vi "State Machine.vi"(0 "private data":T1={"instruction target"=refnum, "channels"=[], "measure state"=enum."Uninitialized", "rx output divider"=enum."1", "equalization mode"=enum."DFE", "rx internal data width"=enum."32 Bit", "BER floor"=0.0, "number of points completed"=0, "rx output divider configured?"=FALSE, "equalization mode configured?"=FALSE, "rx data width configured?"=FALSE}, 5 "requested number of new points":i32, 7 "timeout (100 ms)":dbl=0.1, 11 "error in":errorcluster) -> (4 "private data out":T1={"instruction target"=refnum, "channels"=[], "measure state"=enum."Uninitialized", "rx output divider"=enum."1", "equalization mode"=enum."DFE", "rx internal data width"=enum."32 Bit", "BER floor"=0.0, "number of points completed"=0, "rx output divider configured?"=FALSE, "equalization mode configured?"=FALSE, "rx data width configured?"=FALSE}, 6 "retrieved number of new points":i32, 8 "last point measured?":bool, 14 "timed out?":bool, 15 "error out":errorcluster)   [LabVIEW 2015, in "niHighSpeedSerial Eye Scan v1 Host.lvclass"]
doc: "Manages the state of the Eye Scan engine and handles storing of completed measurements and advancing to measure the next point in the scan.\n\n<B>Input Parameters</B>\n\n<B>private data</B> is the class private data input into the VI.\n\n<B>private data.instruction target</B> is the instruction target to use when communicating with the FPGA.\n\n<B>private data.channels</B> is the array of channel information.\n\n<B>private data.channels.instance</B> is the instance of the channel.\n\n<B>private data.channels.channel</B> is the channel object for a particular channel instance.\n\n<B>private data.channels.point iterator</B> is the point iterator which stores the channel's measured points and controls which point to measure next.\n\n<B>private data.measure state</B> maintains the internal state of the Eye Scan class.\nenum values: Uninitialized,Initialized,Ready,Measuring,Finished,Aborted\n\n<B>private data.rx output divider</B> represents the configuration of the receiver output divider. This should match the values configured with RXRATE and RXOUT_DIV.\nenum values: 1,2,4,8,16\n\n<B>private data.equalization mode</B> indicates the Equalization Mode that the lane is using.\nenum values: DFE,LPM\n\n<B>private data.data width</B> is the data width (in bits) of the receiver lane.\nenum values: 16 Bit,20 Bit,32 Bit,40 Bit\n\n<B>private data.BER floor</B> is the minimum Bit Error Rate which may be computed.\n\n<B>private data.number of points completed</B> is the number of points that have been completed so far by Eye Scan.\n\n<B>private data.rx output divider configured?</B> is true if you have configured the RX Output Divider.\n\n<B>private data.equalization mode configured?</B> is true if you have configured the Equalization Mode\n\n<B>private data.data width configured?</B> is true if you have configured the Data Width.\n\n<B>requested number of new points</B> The number of new points to return, assuming that timeout is not reached, the entire scan doesn't complete, and no errors occur.\n\n<B>timeout (100 ms)</B> The amount of time (in seconds) before timing timing out.\nSpecifying '-1' prevents 'timed out' from ever returning true.\n\n<B>error in</B> describes error conditions that occur before this node runs. This input provides standard 'error in' functionality.\n\n<B>Output Parameters</B>\n\n<B>private data out</B> is the class private data output from the VI.\n\n<B>private data out.instruction target</B> is the instruction target to use when communicating with the FPGA.\n\n<B>private data out.channels</B> is the array of channel information.\n\n<B>private data out.channels.instance</B> is the instance of the channel.\n\n<B>private data out.channels.channel</B> is the channel object for a particular channel instance.\n\n<B>private data out.channels.point iterator</B> is the point iterator which stores the channel's measured points and controls which point to measure next.\n\n<B>private data out.measure state</B> maintains the internal state of the Eye Scan class.\nenum values: Uninitialized,Initialized,Ready,Measuring,Finished,Aborted\n\n<B>private data out.rx output divider</B> represents the configuration of the receiver output divider. This should match the values configured with RXRATE and RXOUT_DIV.\nenum values: 1,2,4,8,16\n\n<B>private data out.equalization mode</B> indicates the Equalization Mode that the lane is using.\nenum values: DFE,LPM\n\n<B>private data out.data width</B> is the data width (in bits) of the receiver lane.\nenum values: 16 Bit,20 Bit,32 Bit,40 Bit\n\n<B>private data out.BER floor</B> is the minimum Bit Error Rate which may be computed.\n\n<B>private data out.number of points completed</B> is the number of points that have been completed so far by the Eye Scan algorithm.\n\n<B>private data out.rx output divider configured?</B> is true if you have configured the RX Output Divider.\n\n<B>private data out.equalization mode configured?</B> is true if you have configured the Equalization Mode.\n\n<B>private data out.data width configured?</B> is true if you have configured the Data Width.\n\n<B>retrieved number of new points</B> The number of new points that were retrieved in this call to Measure.\n\n<B>last point measured?</B> returns true if Eye Scan has completed measuring all points that it was configured to measure.\n\n<B>timed out?</B> returns true if at least 'timeout' amount of time has passed.\n\n<B>error out</B> contains error information. This output provides standard 'error out' functionality."
uses:
  <instrlib>/niHighSpeedSerial/Eye Scan/v1/Host/Eye Scan/niHighSpeedSerial Eye Scan v1 Host.lvclass
  <instrlib>/niHighSpeedSerial/Eye Scan/v1/Host/Eye Scan/Private/Private Data.ctl
  <instrlib>/_niInstr/Instruction Framework/v1/Host/Instruction Target/niInstr Instruction Target v1 Host.lvclass
  <instrlib>/niHighSpeedSerial/Eye Scan/v1/Host/Impl/Eye Scan Point Iterator/niHighSpeedSerial Eye Scan Point Iterator v1 Host.lvclass
  <instrlib>/niHighSpeedSerial/Eye Scan/v1/Host/Eye Scan/Private/Channel Data.ctl
  <instrlib>/niHighSpeedSerial/Eye Scan/v1/Host/Impl/Single Point/niHighSpeedSerial Eye Scan Single Point v1 Host.lvclass
  <instrlib>/niHighSpeedSerial/Eye Scan/v1/Host/Eye Scan/Private/Measure State.ctl
  <instrlib>/niHighSpeedSerial/Eye Scan/v1/Host/Common/Public/RX Output Divider.ctl
  <instrlib>/niHighSpeedSerial/Eye Scan/v1/Host/Common/Public/Equalization Mode.ctl
  <instrlib>/niHighSpeedSerial/Eye Scan/v1/Host/Common/Public/Data Width.ctl
  <instrlib>/niHighSpeedSerial/Eye Scan/v1/Host/Common/niHighSpeedSerial Eye Scan Common v1 Host.lvlib
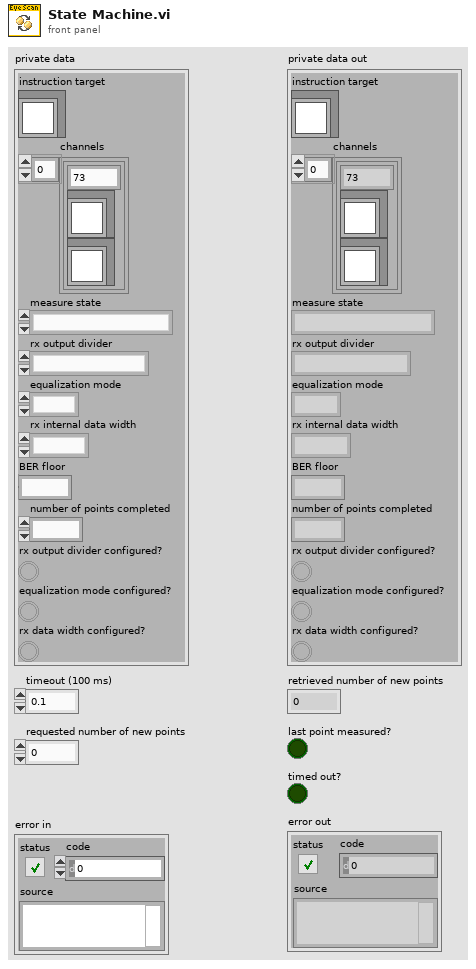
[diagram p1: front panel]
types:
  T1 = typedef "niHighSpeedSerial Eye Scan v1 Host.lvclass/Private Data.ctl" = cluster{"instruction target":refnum<class "niInstr Instruction Target v1 Host.lvclass">, "channels":T2[], "measure state":T3, "rx output divider":T4, "equalization mode":T5, "rx internal data width":T6, "BER floor":dbl, "number of points completed":i32, "rx output divider configured?":bool, "equalization mode configured?":bool, "rx data width configured?":bool}
  T2 = typedef "niHighSpeedSerial Eye Scan v1 Host.lvclass/Channel Data.ctl" = cluster{"instance":u8, "channel":refnum<class "niHighSpeedSerial Eye Scan Single Point v1 Host.lvclass">, "point iterator":refnum<class "niHighSpeedSerial Eye Scan Point Iterator v1 Host.lvclass">}
  T3 = typedef "niHighSpeedSerial Eye Scan v1 Host.lvclass/Measure State.ctl" = enum16{"Uninitialized", "Initialized", "Ready", "Measuring", "Finished", "Aborted"}
  T4 = typedef "niHighSpeedSerial Eye Scan Common v1 Host.lvlib/RX Output Divider.ctl" = enum16{"1", "2", "4", "8", "16"}
  T5 = typedef "niHighSpeedSerial Eye Scan Common v1 Host.lvlib/Equalization Mode.ctl" = enum16{"DFE", "LPM"}
  T6 = typedef "niHighSpeedSerial Eye Scan Common v1 Host.lvlib/Data Width.ctl" = enum16{"16 Bit", "20 Bit", "32 Bit", "40 Bit"}
  T7 = typedef "niHighSpeedSerial Eye Scan Common v1 Host.lvlib/Point Offsets.ctl" = cluster{"horizontal offset":i16, "vertical offset":i8}
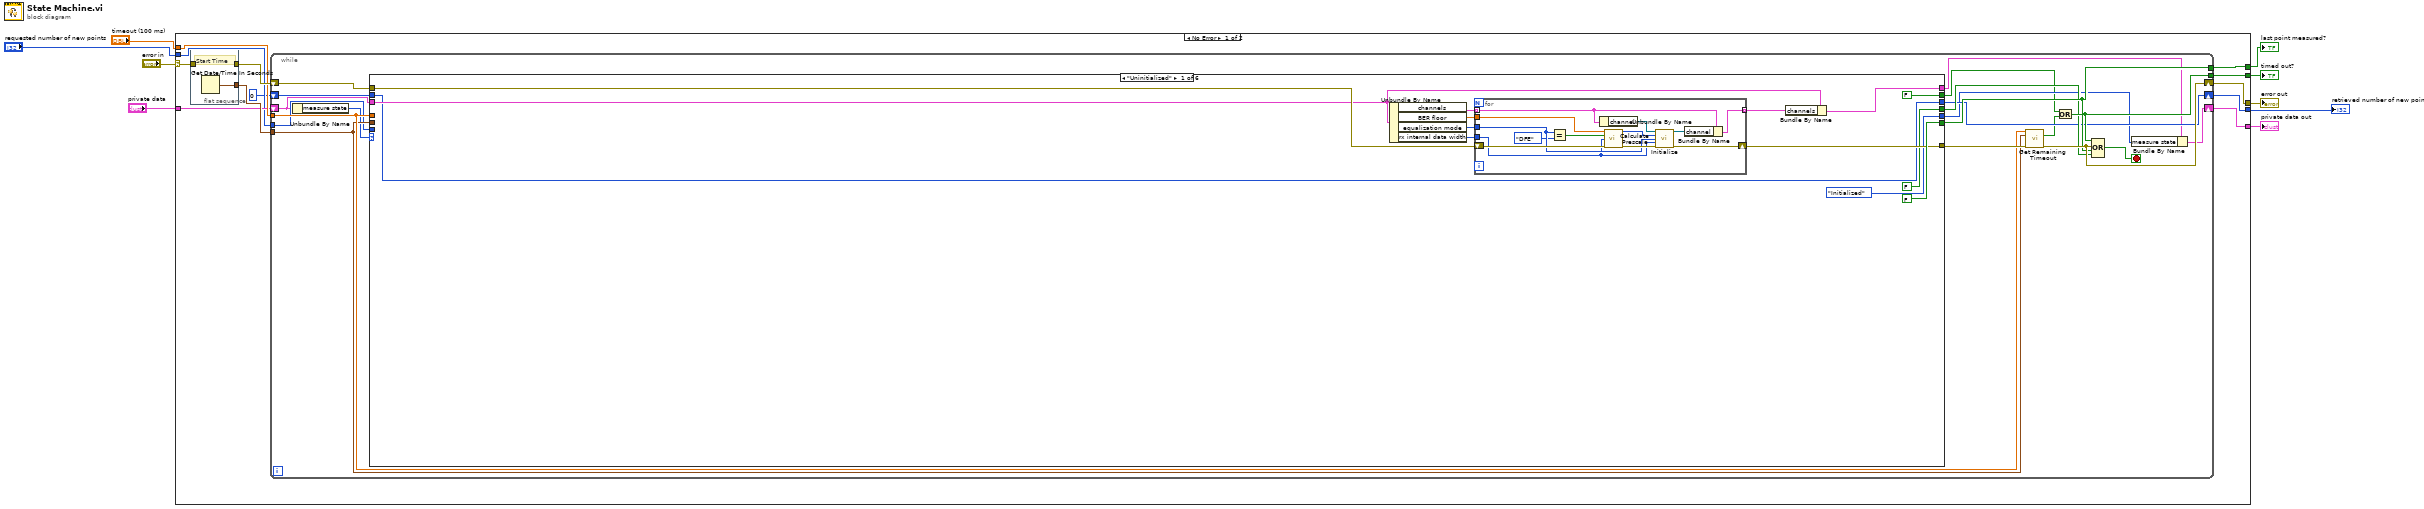
[diagram p0: block diagram]
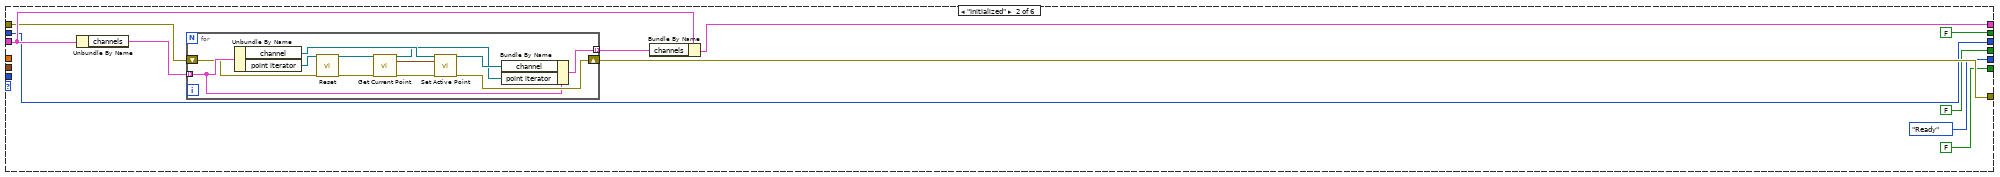
[diagram p2: hidden frame]
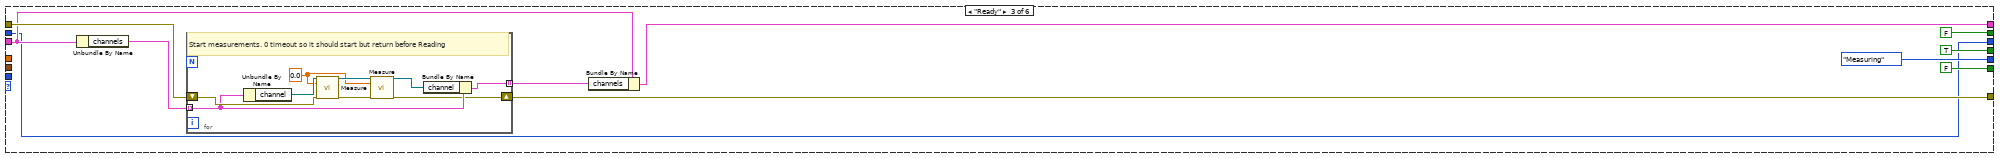
[diagram p3: hidden frame]
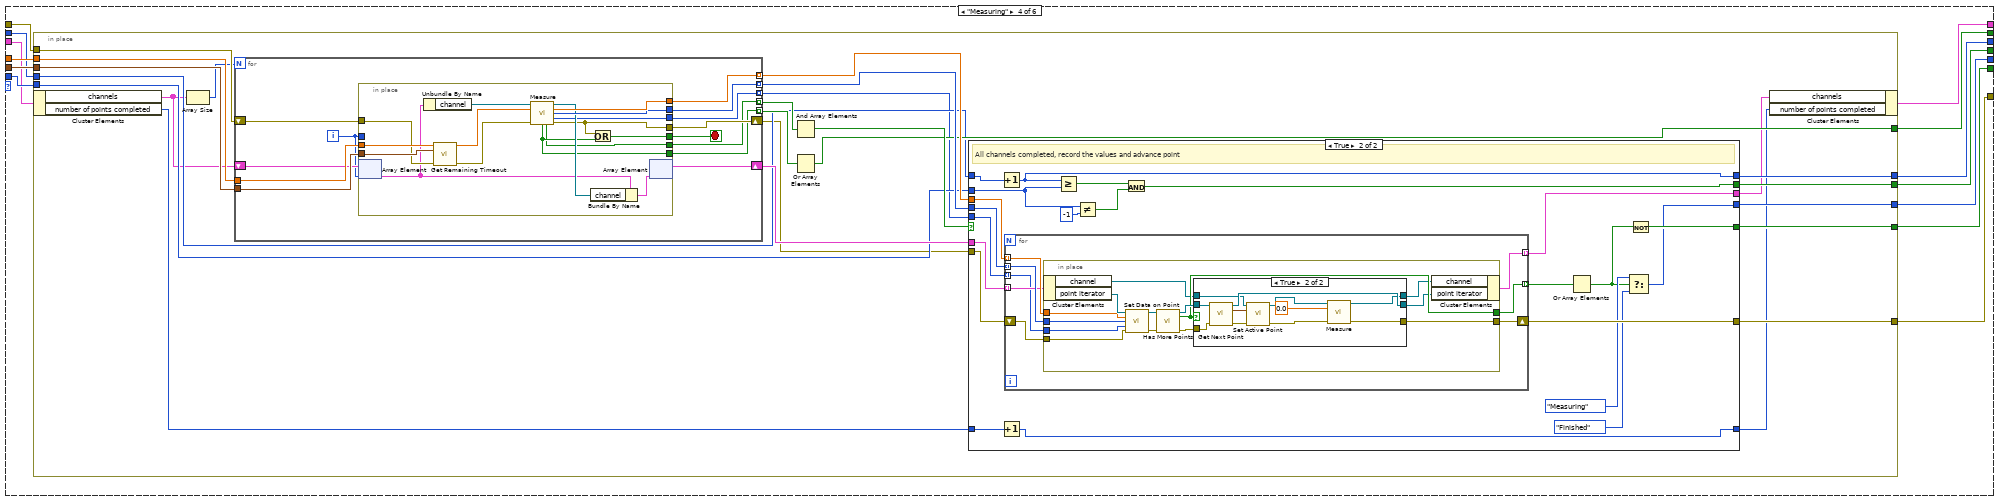
[diagram p4: hidden frame]
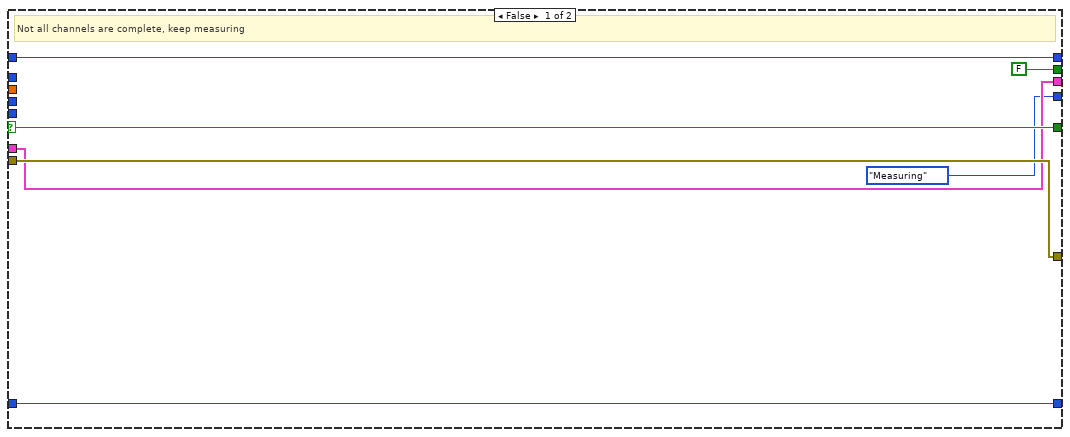
[diagram p5: hidden frame]
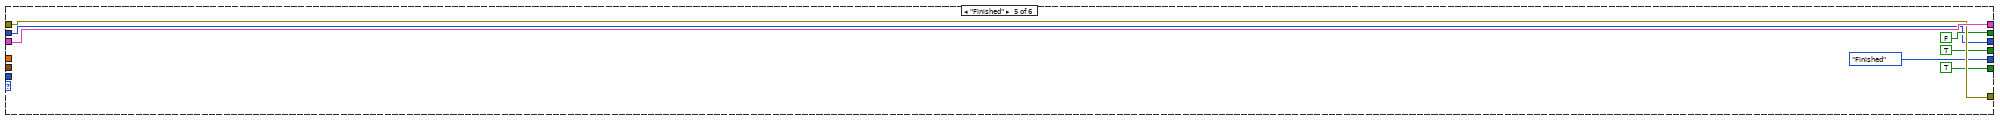
[diagram p7: hidden frame]
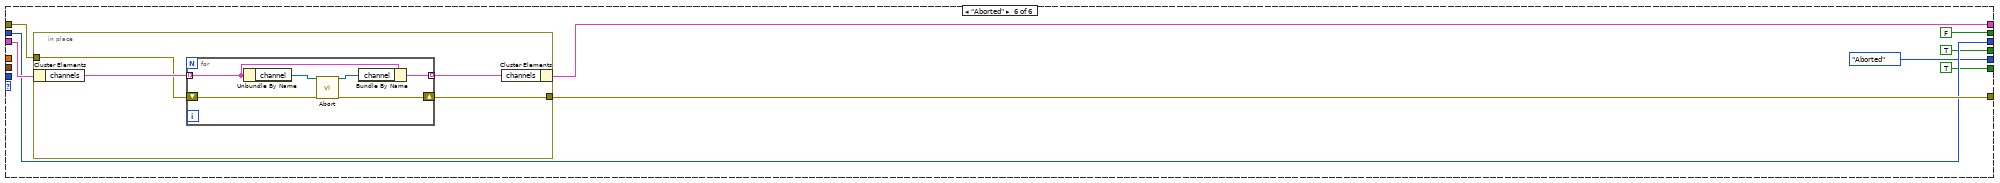
[diagram p8: hidden frame]
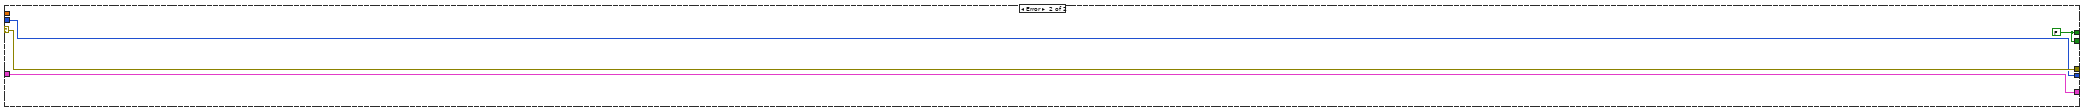
[diagram p9: hidden frame]
diagram:
  n1 = case shown="No Error" "error in" {
    selector: "error in" -> [w20 w272]
    tunnel: "timeout (100 ms)" -> [w18 _]
    tunnel: [w10 w273] -> w7
    tunnel: "private data" -> [w15 w273]
    tunnel: [w16 w272] -> w5
    tunnel: [w17 w271] -> w4
    tunnel: [w14 w271] -> w3
    tunnel: "requested number of new points" -> [w13 w270]
    tunnel: [w11 w270] -> w1
    frame No Error {
      n2 = flat-sequence {
        tunnel: w20 -> [w269]
        tunnel: [w269] -> w19
        tunnel: [w268] -> w21
        frame #0 {
          # "Start Time"
          n3 = Get Date/Time In Seconds() -> (seconds since 1Jan1904=w268:timestamp)
        }
      }
      n4 = while {
        tunnel: w21 -> [w32]
        shift-right: [w37] -> w16
        shift-left: w19 -> [w40]
        tunnel: w18 -> [w33]
        tunnel: [w36] -> w17
        tunnel: [w35] -> w14
        tunnel: w13 -> [w31]
        shift-right: [w29] -> w11
        shift-left: 0 ("Requested Number of Points") -> [w30]
        shift-right: [w24] -> w10
        shift-left: w15 -> [w28]
        stop <- w38 stop-if-true
        n5 = Unbundle By Name(w28) -> ("measure state"=w27:T3)
        n6 = case shown="\"Uninitialized\"" w27 {
          tunnel: w40 -> [w52 w68 w96 w121 w247 w256]
          tunnel: [w51 w77 w95 w119 w247 w255] -> w39
          tunnel: [FALSE ("done") FALSE ("done") FALSE ("done") w120 TRUE ("done") TRUE ("done")] -> w36
          tunnel: [FALSE ("done") FALSE ("done") FALSE ("done") w117 FALSE ("done") FALSE ("done")] -> w22
          tunnel: w28 -> [w49 w72 w94 w112 w248 w257]
          tunnel: [Measure_State."Initialized" ("Measure State") Measure_State."Ready" ("Measure State") Measure_State."Measuring" ("Measure State") w118 Measure_State."Finished" ("Measure State") Measure_State."Aborted" ("Measure State")] -> w25
          tunnel: [w48 w71 w92 w111 w248 w249] -> w26
          tunnel: [FALSE ("done") FALSE ("done") TRUE ("done") w113 TRUE ("done") TRUE ("done")] -> w34
          tunnel: w33 -> [_ _ _ w123 _ _]
          tunnel: w32 -> [_ _ _ w122 _ _]
          tunnel: w31 -> [_ _ _ w115 _ _]
          tunnel: w30 -> [w44 w69 w91 w116 w242 w254]
          tunnel: [w44 w69 w91 w114 w242 w254] -> w29
          frame "Uninitialized" {
            n7 = Unbundle By Name(w49) -> ("channels"=w53:T2[], "BER floor"=w43:dbl, "equalization mode"=w42:T5, "rx internal data width"=w41:T6)
            n8 = for {
              tunnel: w53 -> [w63] mode=indexing
              shift-right: [w67] -> w51
              shift-left: w52 -> [w61]
              tunnel: [w65] -> w47 mode=indexing
              tunnel: w43 -> [w62]
              tunnel: w42 -> [w58]
              tunnel: w41 -> [w55]
              n9 = Equal?(x=w58, y=Equalization_Mode."DFE") -> (x = y?=w56:bool)
              n10 = Unbundle By Name(w63) -> ("channel"=w66:refnum<class "niHighSpeedSerial Eye Scan Single Point v1 Host.lvclass">)
              n11 = call <instrlib>:"Calculate Prescale.vi"("minimum BER"=w62, "in DFE mode?"=w56, "receiver data width"=w55, "error in"=w61) -> ("prescale"=w59:u8, "error out"=w60:errorcluster)  [unwired: 10 in]
              n12 = call-dynamic "Initialize.vi"("eye scan single point"=w66, "prescale"=w59, "equalization mode"=w58, "receiver data width"=w55, "error in"=w60) -> ("eye scan single point out"=w64:refnum<class "niHighSpeedSerial Eye Scan Single Point v1 Host.lvclass">, "error out"=w67:errorcluster)  [unwired: 9 in]
              n13 = Bundle By Name(cluster=w63, "channel"=w64) -> (w65:T2)
            }
            n14 = Bundle By Name(cluster=w49, "channels"=w47) -> (w48:T1)
          }
          frame "Initialized" {
            n15 = Unbundle By Name(w72) -> ("channels"=w78:T2[])
            n16 = for {
              tunnel: w78 -> [w88] mode=indexing
              shift-right: [w90] -> w77
              shift-left: w68 -> [w85]
              tunnel: [w86] -> w70 mode=indexing
              n17 = Unbundle By Name(w88) -> ("channel"=w89:refnum<class "niHighSpeedSerial Eye Scan Single Point v1 Host.lvclass">, "point iterator"=w84:refnum<class "niHighSpeedSerial Eye Scan Point Iterator v1 Host.lvclass">)
              n18 = call-dynamic "Reset.vi"("eye scan point iterator"=w84, "error in"=w85) -> ("eye scan point iterator out"=w83:refnum<class "niHighSpeedSerial Eye Scan Point Iterator v1 Host.lvclass">, "error out"=w82:errorcluster)  [unwired: 12 in]
              n19 = call-dynamic "Get Current Point.vi"("eye scan point iterator"=w83, "error in"=w82) -> ("eye scan point iterator out"=w81:refnum<class "niHighSpeedSerial Eye Scan Point Iterator v1 Host.lvclass">, "current point"=w80:T7, "error out"=w79:errorcluster)  [unwired: 11 in]
              n20 = call-dynamic "Set Active Point.vi"("eye scan single point"=w89, "active point"=w80, "error in"=w79) -> ("eye scan single point out"=w87:refnum<class "niHighSpeedSerial Eye Scan Single Point v1 Host.lvclass">, "error out"=w90:errorcluster)  [unwired: 11 in]
              n21 = Bundle By Name(cluster=w88, "channel"=w87, "point iterator"=w81) -> (w86:T2)
            }
            n22 = Bundle By Name(cluster=w72, "channels"=w70) -> (w71:T1)
          }
          frame "Ready" {
            n23 = Unbundle By Name(w94) -> ("channels"=w97:T2[])
            n24 = for {
              tunnel: w97 -> [w108] mode=indexing
              shift-right: [w103] -> w95
              shift-left: w96 -> [w110]
              tunnel: [w107] -> w93 mode=indexing
              w102 = 0.0 ("Timeout (100 ms)")
              # "Start measurements. 0 timeout so it should start but return before Reading"
              n25 = Unbundle By Name(w108) -> ("channel"=w109:refnum<class "niHighSpeedSerial Eye Scan Single Point v1 Host.lvclass">)
              n26 = call-dynamic "Measure.vi"("eye scan single point"=w109, "timeout (100 ms)"=w102, "error in"=w110) -> ("eye scan single point out"=w106:refnum<class "niHighSpeedSerial Eye Scan Single Point v1 Host.lvclass">, "error out"=w105:errorcluster)  [unwired: 6 in, 5 out]
              n27 = call-dynamic "Measure.vi"("eye scan single point"=w106, "timeout (100 ms)"=w102, "error in"=w105) -> ("eye scan single point out"=w104:refnum<class "niHighSpeedSerial Eye Scan Single Point v1 Host.lvclass">, "error out"=w103:errorcluster)  [unwired: 6 in, 5 out]
              n28 = Bundle By Name(cluster=w108, "channel"=w104) -> (w107:T2)
            }
            n29 = Bundle By Name(cluster=w94, "channels"=w93) -> (w92:T1)
          }
          frame "Measuring" {
            n30 = in-place {
              in-place-border: w123 -> [w147]
              in-place-border: w122 -> [w146]
              in-place-border: w121 -> [w145]
              in-place-border: [w139] -> w120
              in-place-border: [w137] -> w119
              in-place-border: [w136] -> w118
              in-place-border: [w135] -> w117
              in-place-border: w116 -> [w134]
              in-place-border: w115 -> [w133]
              in-place-border: [w132] -> w114
              in-place-border: [w131] -> w113
              n31 = in-place-cluster #1(w112) -> ("channels"=w125:T2[], "number of points completed"=w130:i32)
              n32 = Array Size(array=w125) -> (size(s)=w124:i32)
              n33 = for {
                N: w124 -> [_]
                tunnel: w147 -> [w225]
                tunnel: w146 -> [w224]
                tunnel: [w218] -> w143 mode=indexing
                tunnel: [w217] -> w144 mode=indexing
                tunnel: [w222] -> w141 mode=indexing
                tunnel: [w221] -> w140 mode=indexing
                shift-right: [w219] -> w127
                shift-left: w145 -> [w223]
                tunnel: [w216] -> w126 mode=indexing
                shift-right: [w213] -> w138
                shift-left: w125 -> [w215]
                i -> [w214]
                stop <- w220 stop-if-true
                n34 = in-place {
                  in-place-border: w225 -> [w241]
                  in-place-border: w224 -> [w240]
                  in-place-border: w223 -> [w239]
                  in-place-border: [w236] -> w222
                  in-place-border: [w235] -> w221
                  in-place-border: [w232] -> w220
                  in-place-border: [w231] -> w219
                  in-place-border: [w230] -> w218
                  in-place-border: [w229] -> w217
                  in-place-border: [w228] -> w216
                  in-place-border: w214 -> [_]
                  n35 = in-place-array #2(w215, w214) -> (w227:T2)
                  n36 = Unbundle By Name(w227) -> ("channel"=w234:refnum<class "niHighSpeedSerial Eye Scan Single Point v1 Host.lvclass">)
                  n37 = call <instrlib>:"Get Remaining Timeout.vi"("timeout (100 ms)"=w241, "start time"=w240, "error in"=w239) -> ("remaining timeout"=w237:dbl, "error out"=w238:errorcluster)  [unwired: 10 in, 1 out]
                  n38 = call-dynamic "Measure.vi"("eye scan single point"=w234, "timeout (100 ms)"=w237, "error in"=w238) -> ("eye scan single point out"=w233:refnum<class "niHighSpeedSerial Eye Scan Single Point v1 Host.lvclass">, "bit error ratio"=w236:dbl, "sample count"=w235:u64, "error count"=w228:u64, "timed out?"=w230:bool, "done?"=w229:bool, "error out"=w231:errorcluster)  [unwired: 6 in]
                  n39 = Bundle By Name(cluster=w227, "channel"=w233) -> (w226:T2)
                  n40 = Or(x=w231, y=w230) -> (x .or. y?=w232:bool)
                  n41 = in-place-array #2(w226) -> (w213:T2[])  [unwired: 1 out]
                }
              }
              n42 = And Array Elements(Boolean array=w144) -> (logical AND=w142:bool)
              n43 = Or Array Elements(Boolean array=w143) -> (logical OR=w135:bool)
              n44 = case shown="True" w142 {
                selector: w142 -> [w154 _]
                tunnel: w141 -> [_ w174]
                tunnel: w140 -> [_ w173]
                tunnel: [w154 w172] -> w139
                tunnel: w138 -> [w152 w176]
                tunnel: [w153 w168] -> w137
                tunnel: w127 -> [w153 w175]
                tunnel: [w152 w169] -> w129
                tunnel: [Measure_State."Measuring" ("Measure State") w164] -> w136
                tunnel: w134 -> [w149 w171]
                tunnel: w133 -> [_ w162]
                tunnel: [w149 w170] -> w132
                tunnel: [FALSE w158] -> w131
                tunnel: w130 -> [w148 w156]
                tunnel: [w148 w157] -> w128
                tunnel: w126 -> [_ w155]
                frame False {
                  # "Not all channels are complete, keep measuring"
                }
                frame True {
                  # "All channels completed, record the values and advance point"
                  n45 = Increment(x=w171) -> (x+1=w170:i32)
                  n46 = Increment(x=w156) -> (x+1=w157:i32)
                  n47 = for {
                    tunnel: w176 -> [w179] mode=indexing
                    tunnel: [w178] -> w169 mode=indexing
                    shift-right: [w181] -> w168
                    shift-left: w175 -> [w184]
                    tunnel: w174 -> [w183] mode=indexing
                    tunnel: w173 -> [w182] mode=indexing
                    tunnel: [w180] -> w167 mode=indexing
                    tunnel: w155 -> [w177] mode=indexing
                    n48 = in-place {
                      in-place-border: w184 -> [w198]
                      in-place-border: w183 -> [w185]
                      in-place-border: w182 -> [w186]
                      in-place-border: [w193] -> w181
                      in-place-border: [w192] -> w180
                      in-place-border: w177 -> [w187]
                      n49 = in-place-cluster #3(w179) -> ("channel"=w191:refnum<class "niHighSpeedSerial Eye Scan Single Point v1 Host.lvclass">, "point iterator"=w188:refnum<class "niHighSpeedSerial Eye Scan Point Iterator v1 Host.lvclass">)
                      n50 = call-dynamic "Set Data on Point.vi"("eye scan point iterator"=w188, "bit error ratio"=w185, "sample count"=w186, "error count"=w187, "error in"=w198) -> ("eye scan point iterator out"=w197:refnum<class "niHighSpeedSerial Eye Scan Point Iterator v1 Host.lvclass">, "error out"=w196:errorcluster)  [unwired: 9 in]
                      n51 = call-dynamic "Has More Points.vi"("eye scan point iterator"=w197, "error in"=w196) -> ("eye scan point iterator out"=w194:refnum<class "niHighSpeedSerial Eye Scan Point Iterator v1 Host.lvclass">, "has more points?"=w192:bool, "error out"=w195:errorcluster)  [unwired: 11 in]
                      n52 = case shown="True" w192 {
                        tunnel: w195 -> [w201 w210]
                        tunnel: [w201 w209] -> w193
                        tunnel: [w199 w208] -> w189
                        tunnel: w194 -> [w199 w207]
                        tunnel: w191 -> [w200 w203]
                        tunnel: [w200 w202] -> w190
                        frame False {
                        }
                        frame True {
                          n53 = call-dynamic "Get Next Point.vi"("eye scan point iterator"=w207, "error in"=w210) -> ("eye scan point iterator out"=w208:refnum<class "niHighSpeedSerial Eye Scan Point Iterator v1 Host.lvclass">, "next point"=w212:T7, "error out"=w211:errorcluster)  [unwired: 11 in]
                          n54 = call-dynamic "Set Active Point.vi"("eye scan single point"=w203, "active point"=w212, "error in"=w211) -> ("eye scan single point out"=w206:refnum<class "niHighSpeedSerial Eye Scan Single Point v1 Host.lvclass">, "error out"=w205:errorcluster)  [unwired: 11 in]
                          n55 = call-dynamic "Measure.vi"("eye scan single point"=w206, "timeout (100 ms)"=0.0 ("Timeout (100 ms)"), "error in"=w205) -> ("eye scan single point out"=w202:refnum<class "niHighSpeedSerial Eye Scan Single Point v1 Host.lvclass">, "error out"=w209:errorcluster)  [unwired: 6 in, 5 out]
                        }
                      }
                      n56 = in-place-cluster #3("channel"=w190, "point iterator"=w189) -> (w178:T2)
                    }
                  }
                  n57 = Greater Or Equal?(x=w170, y=w162) -> (x >= y?=w160:bool)
                  n58 = Not Equal?(x=w162, y=-1) -> (x != y?=w159:bool)
                  n59 = And(x=w160, y=w159) -> (x .and. y?=w158:bool)
                  n60 = Or Array Elements(Boolean array=w167) -> (logical OR=w163:bool)
                  n61 = Select(t=Measure_State."Measuring" ("Measure State"), s=w163, f=Measure_State."Finished" ("Measure State")) -> (s? t:f=w164:T3)
                  n62 = Not(x=w163) -> (.not. x?=w172:bool)
                }
              }
              n63 = in-place-cluster #1("channels"=w129, "number of points completed"=w128) -> (w111:T1)
            }
          }
          frame "Finished" {
          }
          frame "Aborted" {
            n64 = in-place {
              in-place-border: w256 -> [w259]
              in-place-border: [w258] -> w255
              n65 = in-place-cluster #4(w257) -> ("channels"=w261:T2[])
              n66 = for {
                tunnel: w261 -> [w264] mode=indexing
                shift-right: [w265] -> w258
                shift-left: w259 -> [w266]
                tunnel: [w262] -> w260 mode=indexing
                n67 = Unbundle By Name(w264) -> ("channel"=w267:refnum<class "niHighSpeedSerial Eye Scan Single Point v1 Host.lvclass">)
                n68 = call-dynamic "Abort.vi"("eye scan single point"=w267, "error in"=w266) -> ("eye scan single point out"=w263:refnum<class "niHighSpeedSerial Eye Scan Single Point v1 Host.lvclass">, "error out"=w265:errorcluster)  [unwired: 12 in]
                n69 = Bundle By Name(cluster=w264, "channel"=w263) -> (w262:T2)
              }
              n70 = in-place-cluster #4("channels"=w260) -> (w249:T1)
            }
          }
        }
        n71 = call <instrlib>:"Get Remaining Timeout.vi"("timeout (100 ms)"=w33, "start time"=w32, "error in"=w39) -> ("timed out?"=w23:bool, "error out"=w37:errorcluster)  [unwired: 10 in, 1 out]
        n72 = Or(x=w22, y=w23) -> (x .or. y?=w35:bool)
        n73 = Compound Arithmetic op=OR(w35, w37, w36, w34) -> (w38:bool)
        n74 = Bundle By Name(cluster=w26, "measure state"=w25) -> (w24:T1)
      }
    }
    frame Error {
      w271 = FALSE ("done")
    }
  }
  "private data out" <- w7
  "error out" <- w5
  "last point measured?" <- w4
  "timed out?" <- w3
  "retrieved number of new points" <- w1
